vi "move_robot.vi"(10 "Distance Moved":dbl, 11 "Robot Properties":T1) -> (2 "Angle Turned":dbl, 3 "Robot Properties Out":T1)   [LabVIEW 2015]
uses:
  Robot.ctl
panel:
  in  "Turn Ratio":dbl=1.0
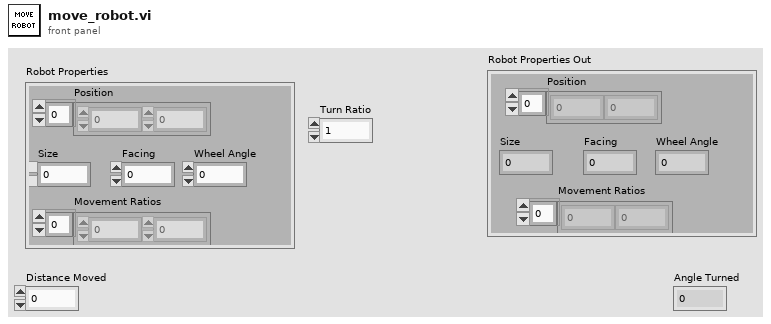
[diagram p1: front panel]
types:
  T1 = typedef "Robot.ctl" = cluster{"Position":dbl[], "Size":dbl, "Facing":dbl, "Movement Ratios":dbl[], "Wheel Angle":dbl}
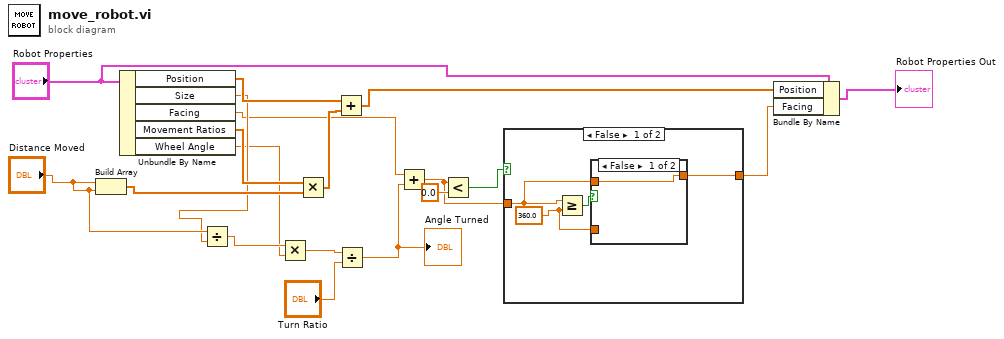
[diagram p0: block diagram]
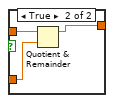
[diagram p2: hidden frame]
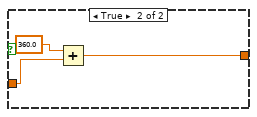
[diagram p3: hidden frame]
diagram:
  n1 = Build Array("Distance Moved", "Distance Moved") -> (w18:dbl[])
  n2 = Unbundle By Name("Robot Properties") -> ("Position"=w16:dbl[], "Size"=w12:dbl, "Facing"=w9:dbl, "Movement Ratios"=w19:dbl[], "Wheel Angle"=w2:dbl)
  n3 = Divide(x="Distance Moved", y=w12) -> (x/y=w11:dbl)
  n4 = Multiply(x=w11, y=w2) -> (x*y=w3:dbl)
  n5 = Multiply(x=w19, y=w18) -> (x*y=w15:dbl[])
  n6 = Add(x=w16, y=w15) -> (x+y=w14:dbl[])
  n7 = Divide(x=w3, y="Turn Ratio") -> (x/y=w1:dbl)
  "Angle Turned" <- w1
  n8 = Add(x=w9, y=w1) -> (x+y=w6:dbl)
  n9 = Less?(x=w6, y=0.0) -> (x < y?=w7:bool)
  n10 = case shown="False" w7 {
    tunnel: w6 -> [w23 w29]
    tunnel: [w21 w28] -> w5
    frame False {
      w22 = 360.0 ("y")
      n11 = Greater Or Equal?(x=w23, y=w22) -> (x >= y?=w20:bool)
      n12 = case shown="False" w20 {
        tunnel: w23 -> [w24 w27]
        tunnel: w22 -> [_ w26]
        tunnel: [w24 w25] -> w21
        frame False {
        }
        frame True {
          n13 = Quotient & Remainder(x=w27, y=w26) -> (x-y*floor(x/y)=w25:dbl)  [unwired: 1 out]
        }
      }
    }
    frame True {
      n14 = Add(x=360.0, y=w29) -> (x+y=w28:dbl)
    }
  }
  n15 = Bundle By Name(cluster="Robot Properties", "Position"=w14, "Facing"=w5) -> (→"Robot Properties Out":T1)
